vi "RIB - Shutdown.vi"(0 "Limits File Path":path, 5 "Results File Path":path, 11 "error in":errorcluster) -> (4 "Results Data Array":string[][](array[string]), 15 "error out":errorcluster)   [LabVIEW 2024]
doc: "Template test"
uses:
  <vilib>/addons/_JKI Toolkits/State Machine/_JKI_lib_State_Machine.llb/Select State(s)_err__jki_lib_state_machine.vi
  <vilib>/addons/_JKI Toolkits/State Machine/_JKI_lib_State_Machine.llb/Periodic Trigger__ogtk__JKI-SM__jki_lib_state_machine.vi
  <userlib>/_OpenG.lib/file/file.llb/Strip Path Extension - String__ogtk.vi
  <vilib>/Utility/file.llb/Read Delimited Spreadsheet (string).vi
  <userlib>/_OpenG.lib/appcontrol/appcontrol.llb/openg_application_control.lvlib
  <userlib>/_OpenG.lib/time/time.llb/openg_time.lvlib
  <userlib>/_OpenG.lib/file/file.llb/openg_file.lvlib
  I2C/libMPSSE-I2C.lvlib
  <vilib>/Utility/file.llb/Write Delimited Spreadsheet (string).vi
panel:
  in  "Exit":bool
  # "Shutdown"
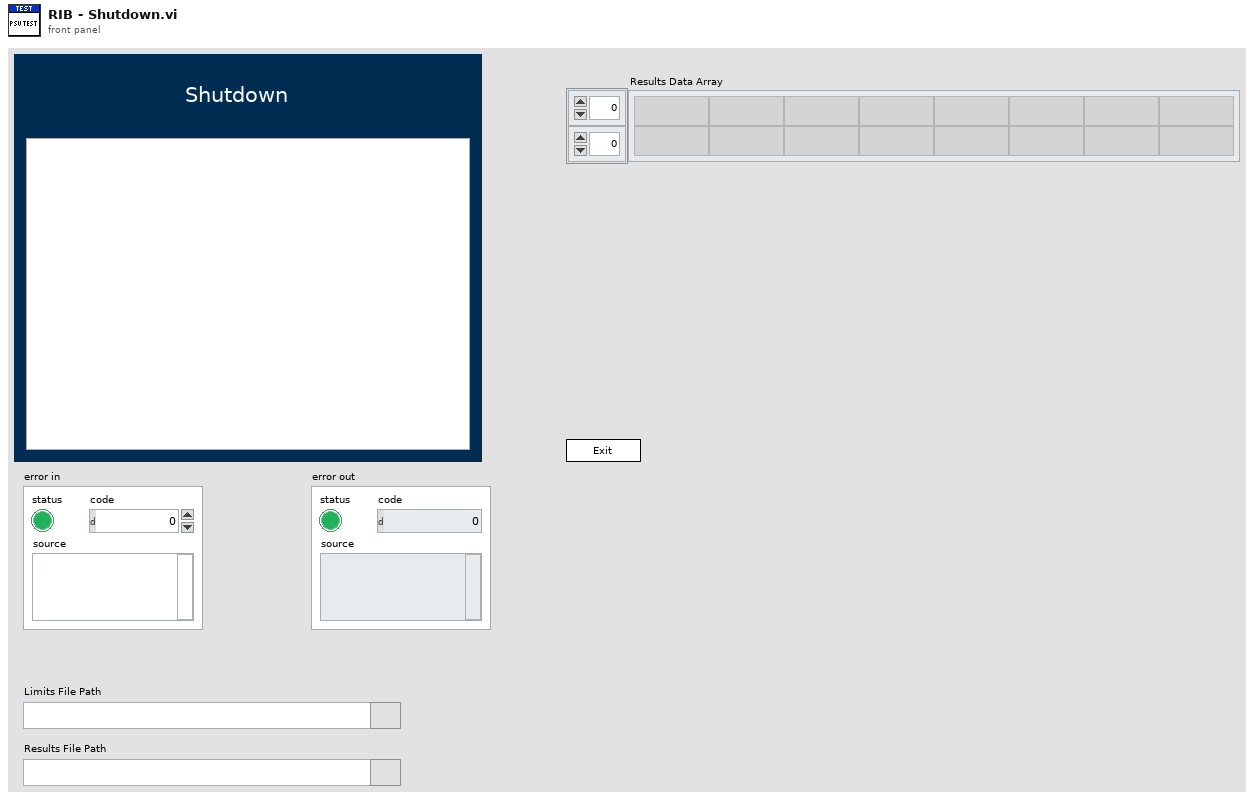
[diagram p1: front panel]
types:
  T1 = enum32{"Invalid", "Standard", "Closed", "Hidden", "Minimized", "Maximized"}
  T2 = enum32{"invalid app kind", "Development System", "Run Time System", "Student Edition", "Embedded LabVIEW", "Evaluation", "Custom"}
  T3 = typedef "FGV - Enum" = enum16{"Cleanup", "Get Data", "Open UDP", "Initialise DAQ", "Initialise I2C"}
  T4 = cluster{"Core":cluster{"Current VI Reference":refnum<vi>, "Close Panel on Exit?":bool}, "Limits File Path":path, "Test Limits":string[][], "Results Data Array":string[][], "Results File Path":path}
  T5 = cluster{"Current VI Reference":refnum<vi>, "Close Panel on Exit?":bool}
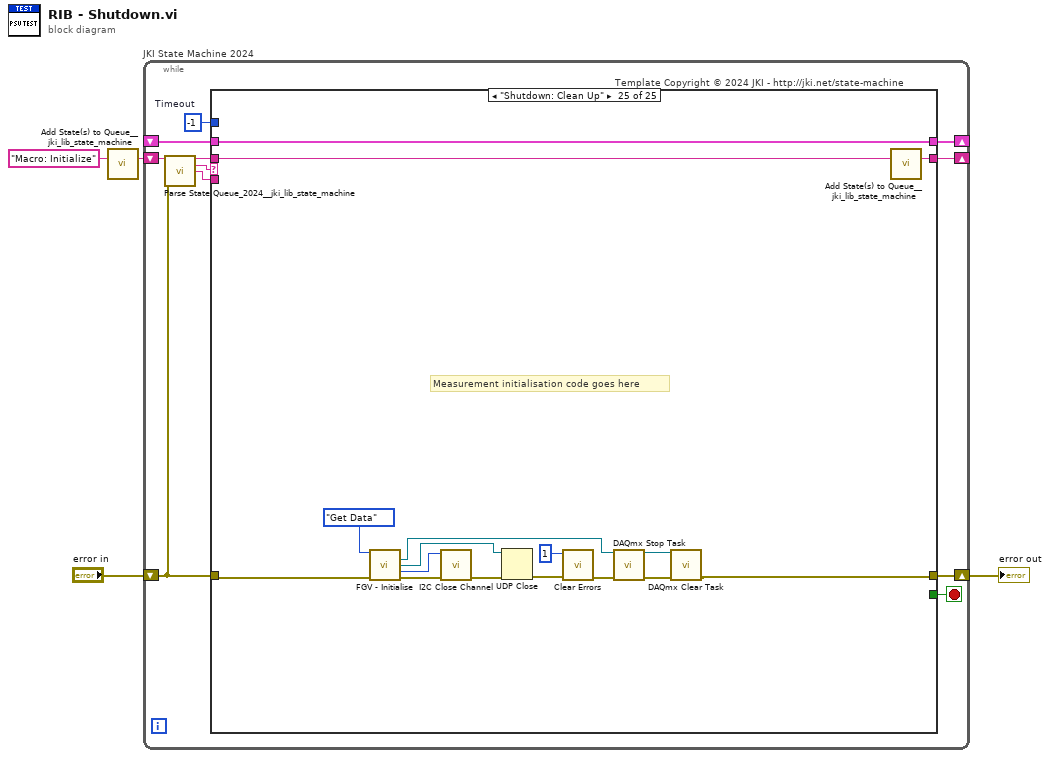
[diagram p0: block diagram]
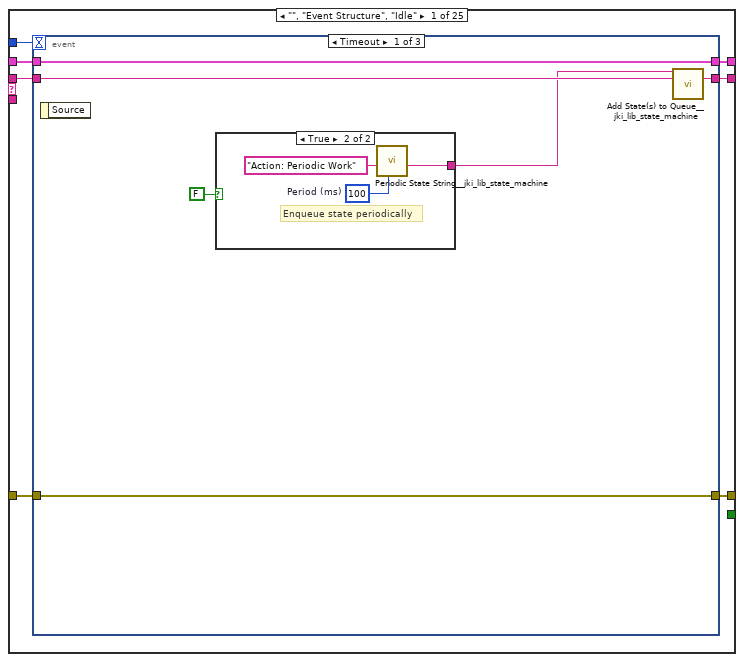
[diagram p2: hidden frame]
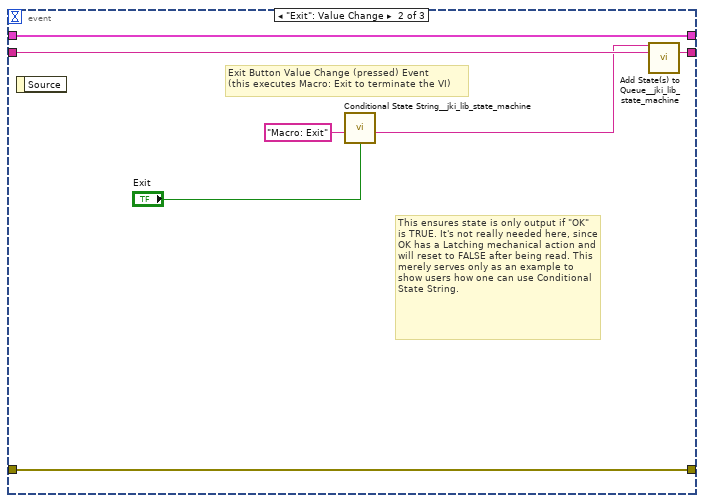
[diagram p4: hidden frame]
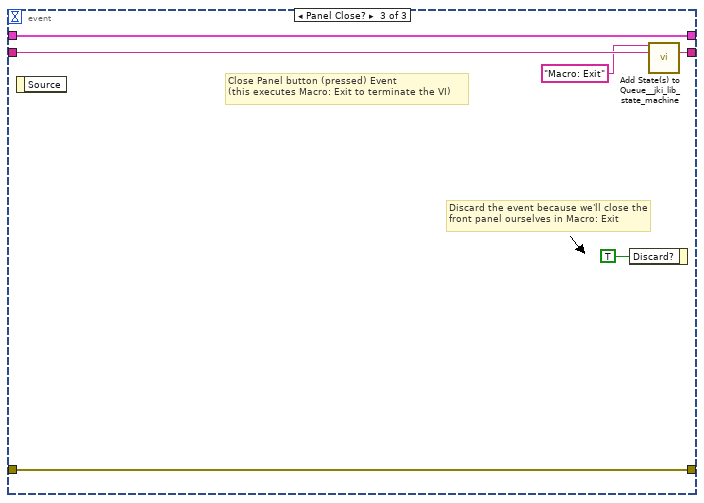
[diagram p5: hidden frame]
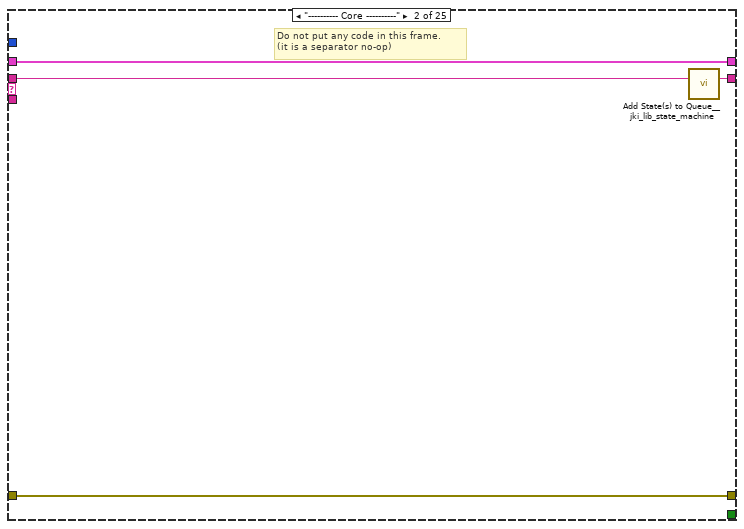
[diagram p6: hidden frame]
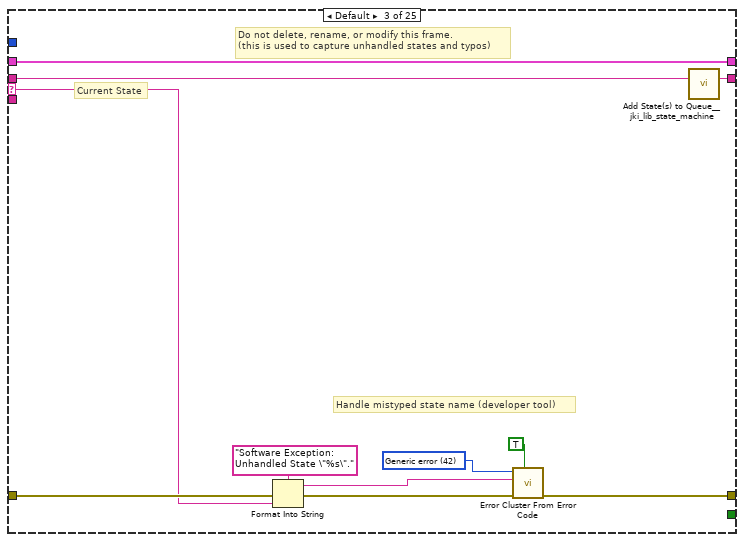
[diagram p7: hidden frame]
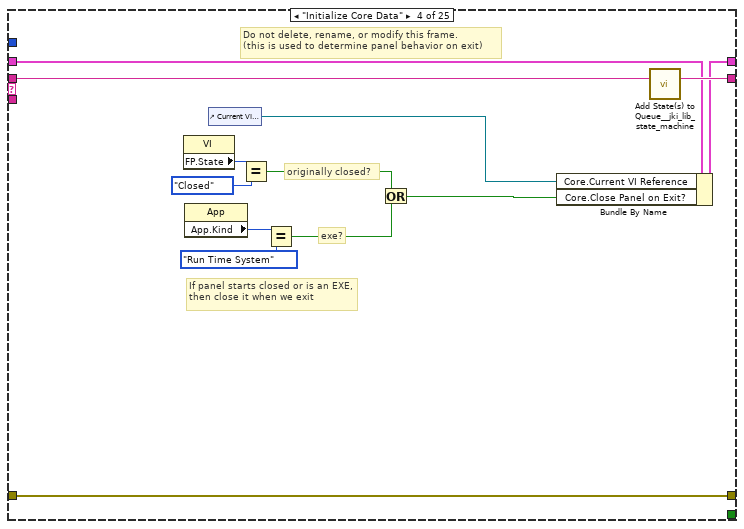
[diagram p8: hidden frame]
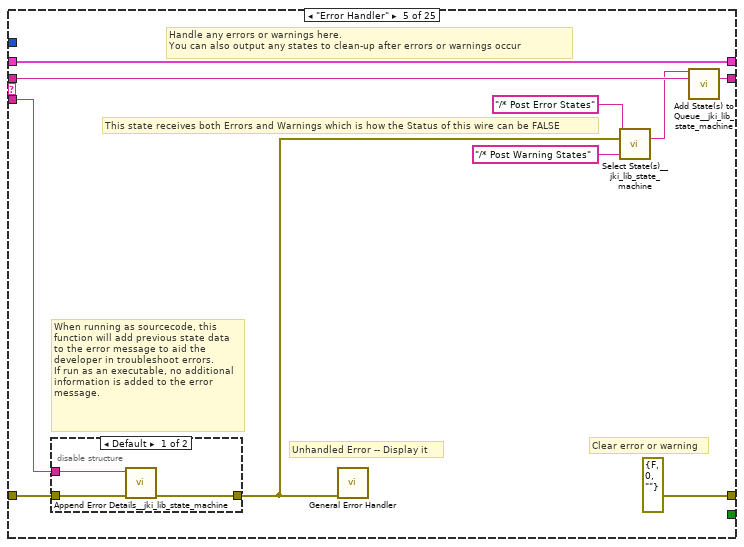
[diagram p9: hidden frame]
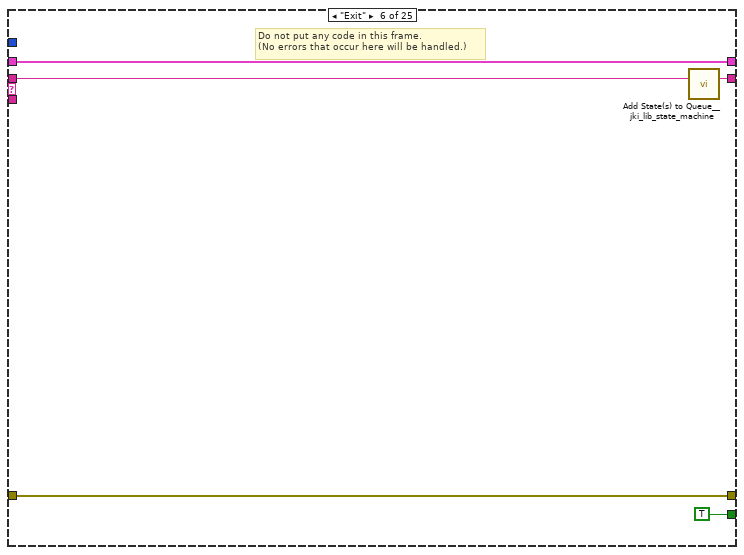
[diagram p11: hidden frame]
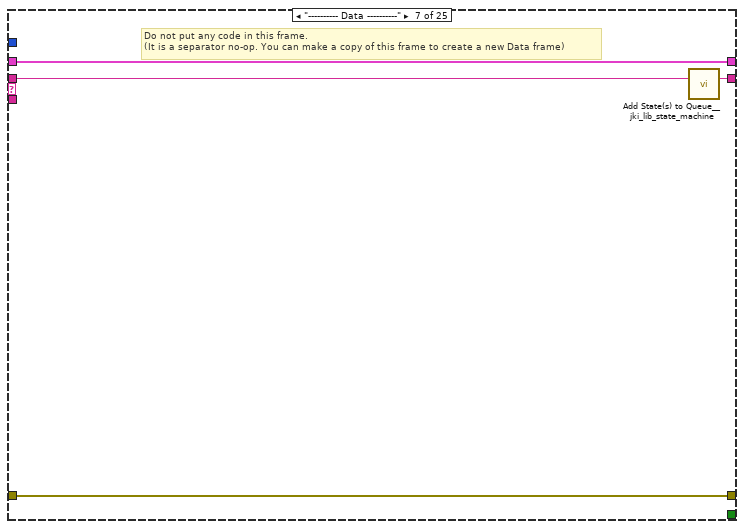
[diagram p12: hidden frame]
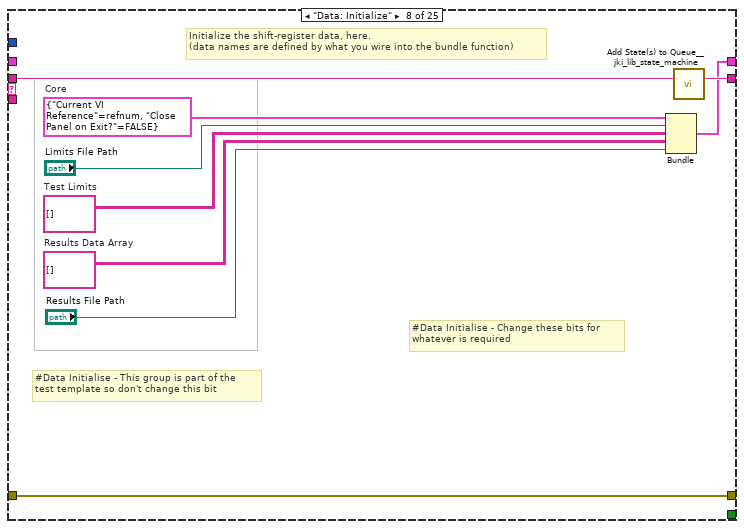
[diagram p13: hidden frame]
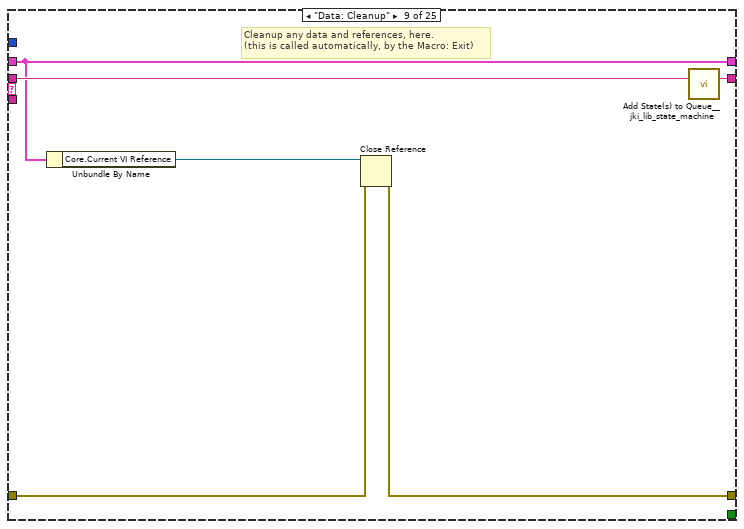
[diagram p14: hidden frame]
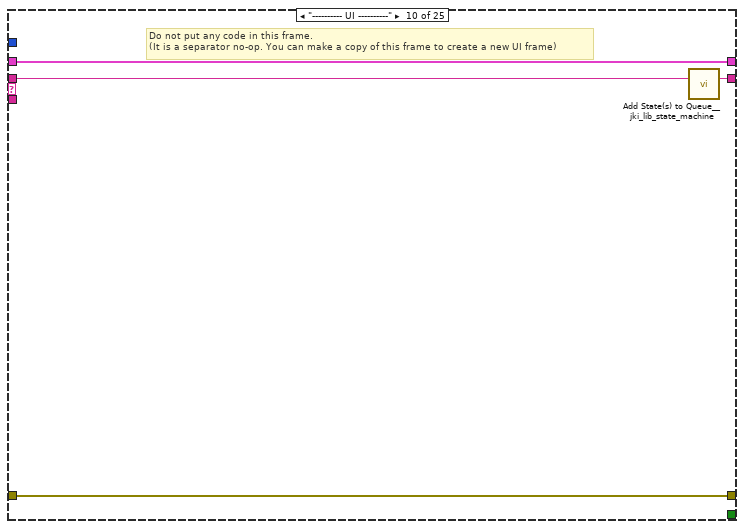
[diagram p15: hidden frame]
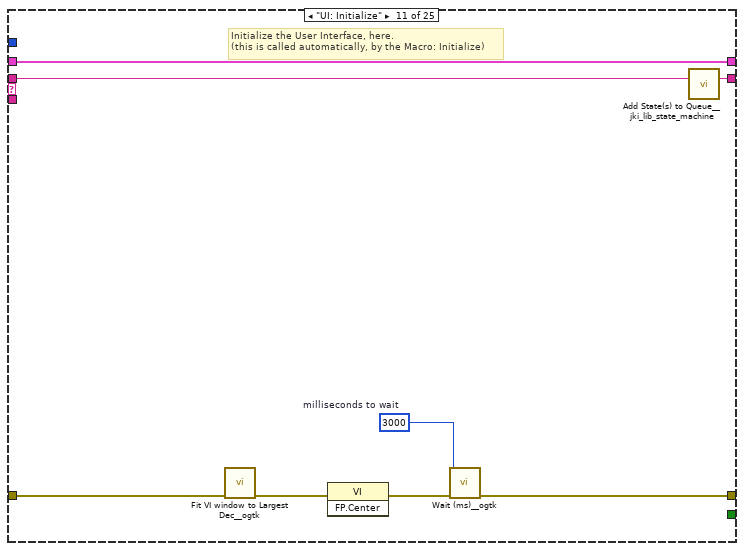
[diagram p16: hidden frame]
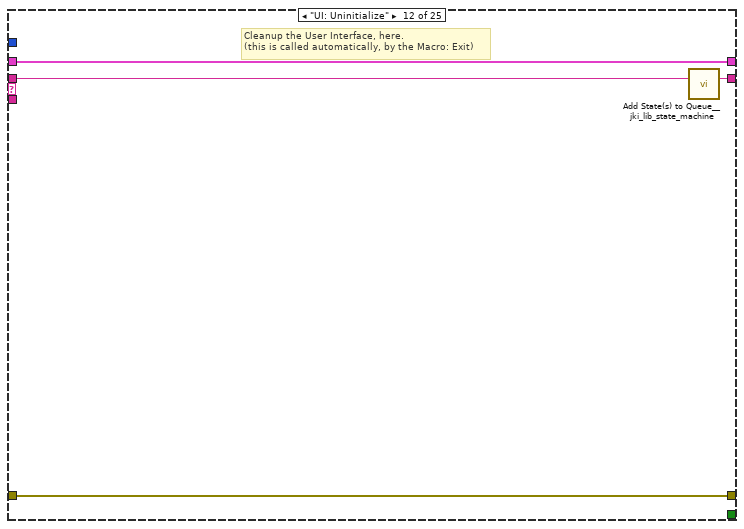
[diagram p17: hidden frame]
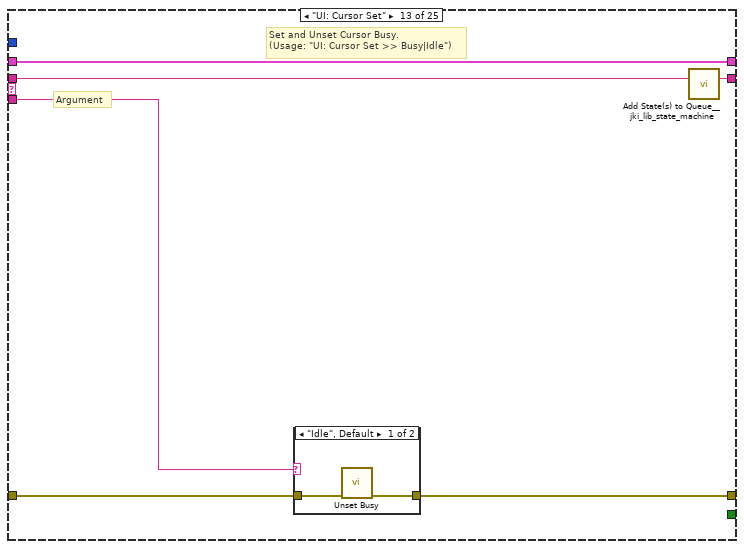
[diagram p18: hidden frame]
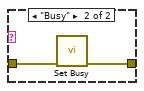
[diagram p19: hidden frame]
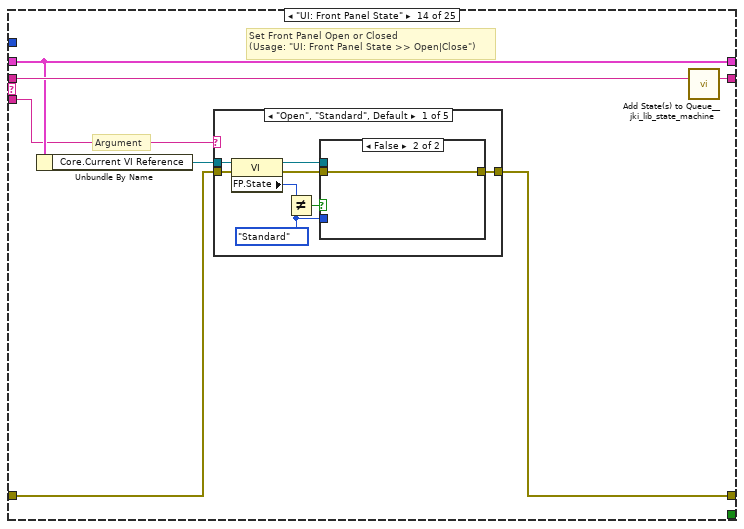
[diagram p20: hidden frame]
diagram:
  n1 = call <vilib>:"Add State(s) to Queue__jki_lib_state_machine.vi"("State(s) in (\"\")"="Macro: Initialize") -> ("States Out"=w4:string)  [unwired: 14 in]
  n2 = while "JKI State Machine 2024" {
    shift-right: [w8] -> _
    shift-left: _ -> [w7]
    shift-right: [w11] -> w1
    shift-left: "error in" -> [w5]
    shift-right: [w10] -> _
    shift-left: w4 -> [w12]
    stop <- w9 stop-if-true
    w6 = -1  # Timeout
    # "Template Copyright © 2024 JKI - http://jki.net/state-machine"
    n3 = call <vilib>:"Parse State Queue_2024__jki_lib_state_machine.vi"("State Queue"=w12, "Error In (no error)"=w5) -> ("Remaining States"=w14:string, "Current State"=w15:string, "Arguments"=w13:string)  [unwired: 11 in]
    n4 = case shown="\"Shutdown: Clean Up\"" w15 {
      selector: w15 -> [_ _ w49 _ _ _ _ _ _ _ _ _ _ _ _ _ _ _ _ _ _ _ _ _ _]
      tunnel: w14 -> [w22 w48 w53 w72 w82 w91 w95 w104 w110 w114 w122 w126 w132 w143 w212 w217 w221 w230 w234 w247 w257 w261 w270 w274 w290]
      tunnel: w13 -> [_ _ _ _ w77 _ _ _ _ _ _ _ w127 w137 _ _ _ _ _ _ _ _ _ _ _]
      tunnel: w7 -> [w20 w45 w51 w65 w79 w89 w92 _ w105 w111 w120 w124 w130 w139 w209 w214 w218 w228 w231 w237 w254 w259 w262 w271 w288]
      tunnel: [w19 w46 w55 w69 errorcluster {"status"=FALSE, "code"=0, "source"=""} ("error out") w88 w93 w101 w106 w112 w118 w123 w128 w140 w210 w215 w219 w225 w232 w235 w255 w258 w263 w272 w276] -> w11
      tunnel: w5 -> [w16 w46 w54 w69 w78 w88 w93 w101 w107 w112 w119 w123 w129 w141 w210 w215 w219 w225 w232 w236 w255 w258 w264 w272 w275]
      tunnel: [w21 w47 w52 w71 w81 w90 w94 w103 w109 w113 w121 w125 w131 w142 w211 w216 w220 w229 w233 w246 w256 w260 w269 w273 w289] -> w10
      tunnel: [_ _ _ _ _ TRUE _ _ _ _ _ _ _ _ _ _ _ _ _ _ _ _ _ _ _] -> w9
      tunnel: [w18 w45 w51 w70 w79 w89 w92 w102 w105 w111 w120 w124 w130 w139 w209 w214 w218 w228 w231 w238 w253 w259 w262 w271 w288] -> w8
      tunnel: w6 -> [w17 _ _ _ _ _ _ _ _ _ _ _ _ _ _ _ _ _ _ _ _ _ _ _ _]
      frame "", "Event Structure", "Idle" {
        n5 = event shown="[0] Timeout" {
          selector: _ -> [_ _ _]
          dyn-events: _ -> [_ _ _]
          timeout: w17 -> [_ _ _]
          tunnel: w22 -> [w28 w38 w44]
          tunnel: [w27 w37 w43] -> w21
          tunnel: w20 -> [w25 w35 w41]
          tunnel: [w26 w36 w42] -> w19
          tunnel: w16 -> [w26 w36 w42]
          tunnel: [w25 w35 w41] -> w18
          event Timeout {
            n6 = event-data() -> ()  [unwired: 1 in, 1 out]
            n7 = case shown="True" FALSE {
              tunnel: [_ w31] -> w24
              frame False {
              }
              frame True {
                w29 = u32 100  # Period (ms)
                # "Enqueue state periodically"
                n8 = call <vilib>:"Periodic State String__jki_lib_state_machine.vi"("Period (ms)"=w29, "State"="Action: Periodic Work") -> ("State Out"=w31:string)  [unwired: 9 in]
              }
            }
            n9 = call <vilib>:"Add State(s) to Queue__jki_lib_state_machine.vi"("State(s) in Front (\"\")"=w24, "State(s) in (\"\")"=w28) -> ("States Out"=w27:string)  [unwired: 13 in]
          }
          event "Exit": Value Change {
            # "This ensures state is only output if \"OK\" is TRUE. It's not really needed here, since OK has a Latching mechanical action and will reset to FALSE after being read. This merely serves only as an example to show users how one can use Conditional State String."
            # "Exit Button Value Change (pressed) Event\n(this executes Macro: Exit to terminate the VI)"
            n10 = event-data() -> ()  [unwired: 1 in, 1 out]
            n11 = call <vilib>:"Conditional State String__jki_lib_state_machine.vi"("Do State(s)?"="Exit", "State"="Macro: Exit") -> ("State Out"=w32:string)  [unwired: 7 in]
            n12 = call <vilib>:"Add State(s) to Queue__jki_lib_state_machine.vi"("State(s) in Front (\"\")"=w32, "State(s) in (\"\")"=w38) -> ("States Out"=w37:string)  [unwired: 13 in]
          }
          event Panel Close? {
            # "Discard the event because we'll close the front panel ourselves in Macro: Exit"
            # "Close Panel button (pressed) Event\n(this executes Macro: Exit to terminate the VI)"
            n13 = event-data() -> ()  [unwired: 1 in, 1 out]
            n14 = event-data("Discard?"=TRUE) -> ()  [unwired: 1 in, 1 out]
            n15 = call <vilib>:"Add State(s) to Queue__jki_lib_state_machine.vi"("State(s) in Front (\"\")"="Macro: Exit", "State(s) in (\"\")"=w44) -> ("States Out"=w43:string)  [unwired: 13 in]
          }
        }
      }
      frame "---------- Core ----------" {
        # "Do not put any code in this frame.\n(it is a separator no-op)"
        n16 = call <vilib>:"Add State(s) to Queue__jki_lib_state_machine.vi"("State(s) in (\"\")"=w48) -> ("States Out"=w47:string)  [unwired: 14 in]
      }
      frame Default {
        w58 = 42 items=["No error", "Argument error", "Memory is full", "Out of zone", "End of file", "File already open", "Generic file I/O error", "File not found", "File permission error", "Disk is full", "Duplicate path", "Too many files open", "System feature not enabled", "Resource file not found", "Cannot add resource", "Resource not found", "Image not found", "Image memory error", "Pen does not exist", "Config type invalid", "Config token not found", "Config parse error", "Config memory error", "Bad external code format", "Bad external code offset", "External code not present", "Null window", "Destroy window error", "Null menu", "Print aborted", "Bad print record", "Print driver error", "Windows error during printing", "Memory error during printing", "Print dialog error", "Generic print error", "Invalid device refnum", "Device not found", "Device parameter error", "Device unit error", "Cannot open device", "Device call aborted", "Generic error", "Cancelled by user", "Object ID too low", "Object ID too high", "Object not in heap", "Unknown heap", "Unknown object (invalid DefProc)", "Unknown object (DefProc not in table)", "Message out of range", "Invalid (null) method", "Unknown message", "Manager call not supported", "Bad address", "Network operation in progress", "Network operation timed out", "Connection is busy", "Network attribute not supported", "Network error", "Address in use", "System out of memory", "Connection aborted", "Connection refused", "Not connected", "Already connected", "Connection closed", "Initialization error (interapplication manager)", "Bad occurrence", "Wait on unbound occurrence handler", "Occurrence queue overflow", "Datalog type conflict", "Unused", "Unrecognized type (interapplication manager)", "Memory corrupt", "Failed to make temporary DLL", "Old CIN version", "Drag socket not found", "Failed to load drop-object", "Failed to register OLE object", "Failed to release OLE object", "Format specifier type mismatch", "Unknown format specifier", "Too few format specifiers", "Too many format specifiers", "Scan failed", "Newer CIN version", "Error converting to variant", "Runtime menu error", "Password tampered", "Variant attribute not found", "Incompatible variant data type", "Event data is not available", "Event Store is not present", "Occurrence is not found", "Event Queue is not created", "Event info is not available", "Refnum passed is NULL", "Error retrieving Class GUID", "Error retrieving CoClass GUID", "Error retrieving TypeLib GUID.", "Bad built application magic bytes.", "Specific driver is different from the specific driver associated with the Logical Name.", "There is no session opened to the class driver.", "Max Error", "MAX - Error with config objects", "MAX - Error loading configuration", "MAX - Group not supported"]
        # "Current State"
        # "Do not delete, rename, or modify this frame.\n(this is used to capture unhandled states and typos)"
        # "Handle mistyped state name (developer tool)"
        n17 = Format Into String(format string="Software Exception: Unhandled State \"%s\"." ("message"), error in=w54, w49) -> (resulting string=w57:string, error out=w56:errorcluster)  [unwired: 1 in]
        n18 = call <vilib>:"Error Cluster From Error Code.vi"("show call chain? (False)"=TRUE, "error in (no error)"=w56, "error message (\"\")"=w57, "error code (0)"=w58) -> ("error out"=w55:errorcluster)  [unwired: 5 in]
        n19 = call <vilib>:"Add State(s) to Queue__jki_lib_state_machine.vi"("State(s) in (\"\")"=w53) -> ("States Out"=w52:string)  [unwired: 14 in]
      }
      frame "Initialize Core Data" {
        # "Do not delete, rename, or modify this frame.\n(this is used to determine panel behavior on exit)"
        # "originally closed?"
        # "exe?"
        # "If panel starts closed or is an EXE, then close it when we exit"
        n20 = property class="VI"() -> ("FP.State"=w62:T1)  [unwired: 2 in, 2 out]
        n21 = property class="App"() -> ("App.Kind"=w68:T2)  [unwired: 2 in, 2 out]
        n22 = control-ref of="Current VI Reference"() -> (w63:refnum<vi>)
        n23 = Equal?(x=w62, y=T1."Closed" ("Front Panel Window:State")) -> (x = y?=w60:bool)
        n24 = Equal?(x=w68, y=T2."Run Time System" ("Application:Kind")) -> (x = y?=w66:bool)
        n25 = Or(x=w60, y=w66) -> (x .or. y?=w64:bool)
        n26 = Bundle By Name(cluster=w65, "Core.Current VI Reference"=w63, "Core.Close Panel on Exit?"=w64) -> (w70:T4)
        n27 = call <vilib>:"Add State(s) to Queue__jki_lib_state_machine.vi"("State(s) in (\"\")"=w72) -> ("States Out"=w71:string)  [unwired: 14 in]
      }
      frame "Error Handler" {
        # "When running as sourcecode, this function will add previous state data to the error message to aid the developer in troubleshoot errors.\nIf run as an executable, no additional information is added to the error message."
        # "This state receives both Errors and Warnings which is how the Status of this wire can be FALSE"
        # "Unhandled Error -- Display it"
        # "Handle any errors or warnings here.\nYou can also output any states to clean-up after errors or warnings occur"
        # "Clear error or warning"
        n28 = disable-structure shown="Default" {
          disable-tunnel: w78 -> [w85 w86]
          disable-tunnel: w77 -> [w84 _]
          disable-tunnel: [w83 w86] -> w76
          frame condition #0 (active) {
            n29 = call <vilib>:"Append Error Details__jki_lib_state_machine.vi"("error in (no error)"=w85, "Previous State and Argument(s)"=w84) -> ("error out"=w83:errorcluster)  [unwired: 9 in]
          }
          frame condition #1 {
          }
        }
        n30 = call <vilib>:"General Error Handler.vi"("error in (no error)"=w76) -> ()  [unwired: 10 in, 5 out]
        n31 = call-poly <vilib>:"Select State(s)__jki_lib_state_machine.vi"("State(s) if True (\"\")"="/* Post Error States", "Select"=w76, "State(s) if False (\"\")"="/* Post Warning States") -> ("States Out"=w74:string)  [unwired: 12 in]
        n32 = call <vilib>:"Add State(s) to Queue__jki_lib_state_machine.vi"("State(s) in Front (\"\")"=w74, "State(s) in (\"\")"=w82) -> ("States Out"=w81:string)  [unwired: 13 in]
      }
      frame "Exit" {
        # "Do not put any code in this frame.\n(No errors that occur here will be handled.)"
        n33 = call <vilib>:"Add State(s) to Queue__jki_lib_state_machine.vi"("State(s) in (\"\")"=w91) -> ("States Out"=w90:string)  [unwired: 14 in]
      }
      frame "---------- Data ----------" {
        # "Do not put any code in this frame.\n(It is a separator no-op. You can make a copy of this frame to create a new Data frame)"
        n34 = call <vilib>:"Add State(s) to Queue__jki_lib_state_machine.vi"("State(s) in (\"\")"=w95) -> ("States Out"=w94:string)  [unwired: 14 in]
      }
      frame "Data: Initialize" {
        w97 = string[][] []  # Results Data Array
        w98 = string[][] []  # Test Limits
        w100 = T5 {"Current VI Reference"=refnum, "Close Panel on Exit?"=FALSE}  # Core
        # "#Data Initialise - Change these bits for\nwhatever is required"
        # "#Data Initialise - This group is part of the\ntest template so don't change this bit"
        # "Initialize the shift-register data, here.\n(data names are defined by what you wire into the bundle function)"
        n35 = Bundle("Core"=w100, "Limits File Path"="Limits File Path", "Test Limits"=w98, "Results Data Array"=w97, "Results File Path"="Results File Path") -> (w102:T4)  [unwired: 1 in]
        n36 = call <vilib>:"Add State(s) to Queue__jki_lib_state_machine.vi"("State(s) in (\"\")"=w104) -> ("States Out"=w103:string)  [unwired: 14 in]
      }
      frame "Data: Cleanup" {
        # "Cleanup any data and references, here.\n(this is called automatically, by the Macro: Exit)"
        n37 = Unbundle By Name(w105) -> ("Core.Current VI Reference"=w108:refnum<vi>)
        n38 = Close Reference(reference=w108, error in (no error)=w107) -> (error out=w106:errorcluster)
        n39 = call <vilib>:"Add State(s) to Queue__jki_lib_state_machine.vi"("State(s) in (\"\")"=w110) -> ("States Out"=w109:string)  [unwired: 14 in]
      }
      frame "---------- UI ----------" {
        # "Do not put any code in this frame.\n(It is a separator no-op. You can make a copy of this frame to create a new UI frame)"
        n40 = call <vilib>:"Add State(s) to Queue__jki_lib_state_machine.vi"("State(s) in (\"\")"=w114) -> ("States Out"=w113:string)  [unwired: 14 in]
      }
      frame "UI: Initialize" {
        w117 = u32 3000  # milliseconds to wait
        # "Initialize the User Interface, here.\n(this is called automatically, by the Macro: Initialize)"
        n41 = call <userlib>:"Fit VI window to Largest Dec__ogtk.vi"("error in (no error)"=w119) -> ("error out"=w115:errorcluster)  [unwired: 5 in, 1 out]
        n42 = invoke class="VI" method="FP.Center"(error in=w115) -> (error out=w116:errorcluster)  [unwired: 2 in, 2 out]
        n43 = call <userlib>:"Wait (ms)__ogtk.vi"("error in (no error)"=w116, "milliseconds to wait"=w117) -> ("error out"=w118:errorcluster)  [unwired: 8 in, 1 out]
        n44 = call <vilib>:"Add State(s) to Queue__jki_lib_state_machine.vi"("State(s) in (\"\")"=w122) -> ("States Out"=w121:string)  [unwired: 14 in]
      }
      frame "UI: Uninitialize" {
        # "Cleanup the User Interface, here.\n(this is called automatically, by the Macro: Exit)"
        n45 = call <vilib>:"Add State(s) to Queue__jki_lib_state_machine.vi"("State(s) in (\"\")"=w126) -> ("States Out"=w125:string)  [unwired: 14 in]
      }
      frame "UI: Cursor Set" {
        # "Argument"
        # "Set and Unset Cursor Busy.\n(Usage: \"UI: Cursor Set >> Busy|Idle\")"
        n46 = case shown="\"Idle\", Default" w127 {
          tunnel: w129 -> [w134 w136]
          tunnel: [w133 w135] -> w128
          frame "Idle", Default {
            n47 = call <vilib>:"Unset Busy.vi"("error in (no error)"=w134) -> ("error out"=w133:errorcluster)  [unwired: 10 in]
          }
          frame "Busy" {
            n48 = call <vilib>:"Set Busy.vi"("error in (no error)"=w136) -> ("error out"=w135:errorcluster)  [unwired: 9 in, 1 out]
          }
        }
        n49 = call <vilib>:"Add State(s) to Queue__jki_lib_state_machine.vi"("State(s) in (\"\")"=w132) -> ("States Out"=w131:string)  [unwired: 14 in]
      }
      frame "UI: Front Panel State" {
        # "Argument"
        # "Set Front Panel Open or Closed\n(Usage: \"UI: Front Panel State >> Open|Close\")"
        n50 = Unbundle By Name(w139) -> ("Core.Current VI Reference"=w138:refnum<vi>)
        n51 = case shown="\"Open\", \"Standard\", Default" w137 {
          tunnel: w141 -> [w149 w164 w175 w188 w201]
          tunnel: [w151 w165 w177 w190 w203] -> w140
          tunnel: w138 -> [w150 w162 w176 w189 w202]
          frame "Open", "Standard", Default {
            w144 = T1."Standard" ("State")
            n52 = property class="VI"(reference=w150, error in=w149) -> (reference out=w147:refnum<vi>, error out=w148:errorcluster, "FP.State"=w146:T1)
            n53 = Not Equal?(x=w146, y=w144) -> (x != y?=w145:bool)
            n54 = case shown="False" w145 {
              tunnel: [w155 w157] -> w151
              tunnel: w148 -> [w154 w157]
              tunnel: w147 -> [w153 _]
              tunnel: w144 -> [w152 _]
              frame True {
                n55 = invoke class="VI" method="FP.Open"(reference=w153, error in=w154, "Activate"=TRUE, "State"=w152) -> (error out=w155:errorcluster)  [unwired: 1 in, 4 out]
              }
              frame False {
              }
            }
          }
          frame "Close", "Closed" {
            n56 = property class="VI"(reference=w162, error in=w164) -> (reference out=w161:refnum<vi>, error out=w163:errorcluster, "FP.State"=w159:T1)
            n57 = Not Equal?(x=w159, y=T1."Closed" ("Front Panel Window:State")) -> (x != y?=w158:bool)
            n58 = case shown="True" w158 {
              tunnel: [w166 w169] -> w165
              tunnel: w163 -> [w166 w168]
              tunnel: w161 -> [_ w167]
              frame False {
              }
              frame True {
                n59 = invoke class="VI" method="FP.Close"(reference=w167, error in=w168) -> (error out=w169:errorcluster)  [unwired: 1 in, 2 out]
              }
            }
          }
          frame "Hidden", "Hide" {
            w170 = T1."Hidden" ("State")
            n60 = property class="VI"(reference=w176, error in=w175) -> (reference out=w173:refnum<vi>, error out=w174:errorcluster, "FP.State"=w172:T1)
            n61 = Not Equal?(x=w172, y=w170) -> (x != y?=w171:bool)
            n62 = case shown="True" w171 {
              tunnel: [w181 w182] -> w177
              tunnel: w174 -> [w180 w182]
              tunnel: w173 -> [w179 _]
              tunnel: w170 -> [w178 _]
              frame True {
                n63 = invoke class="VI" method="FP.Open"(reference=w179, error in=w180, "State"=w178) -> (error out=w181:errorcluster)  [unwired: 2 in, 4 out]
              }
              frame False {
              }
            }
          }
          frame "Minimize", "Minimized" {
            w183 = T1."Minimized" ("State")
            n64 = property class="VI"(reference=w189, error in=w188) -> (reference out=w186:refnum<vi>, error out=w187:errorcluster, "FP.State"=w185:T1)
            n65 = Not Equal?(x=w185, y=w183) -> (x != y?=w184:bool)
            n66 = case shown="True" w184 {
              tunnel: [w194 w195] -> w190
              tunnel: w187 -> [w193 w195]
              tunnel: w186 -> [w192 _]
              tunnel: w183 -> [w191 _]
              frame True {
                n67 = invoke class="VI" method="FP.Open"(reference=w192, error in=w193, "State"=w191) -> (error out=w194:errorcluster)  [unwired: 2 in, 4 out]
              }
              frame False {
              }
            }
          }
          frame "Maximize", "Maximized" {
            w196 = T1."Maximized" ("State")
            n68 = property class="VI"(reference=w202, error in=w201) -> (reference out=w199:refnum<vi>, error out=w200:errorcluster, "FP.State"=w198:T1)
            n69 = Not Equal?(x=w198, y=w196) -> (x != y?=w197:bool)
            n70 = case shown="True" w197 {
              tunnel: [w207 w208] -> w203
              tunnel: w200 -> [w206 w208]
              tunnel: w199 -> [w205 _]
              tunnel: w196 -> [w204 _]
              frame True {
                n71 = invoke class="VI" method="FP.Open"(reference=w205, error in=w206, "State"=w204) -> (error out=w207:errorcluster)  [unwired: 2 in, 4 out]
              }
              frame False {
              }
            }
          }
        }
        n72 = call <vilib>:"Add State(s) to Queue__jki_lib_state_machine.vi"("State(s) in (\"\")"=w143) -> ("States Out"=w142:string)  [unwired: 14 in]
      }
      frame "---------- Macro ----------" {
        # "Do not put any code in this frame.\n(It is a separator no-op. You can make a copy of this frame to create a new Macro frame)"
        n73 = call <vilib>:"Add State(s) to Queue__jki_lib_state_machine.vi"("State(s) in (\"\")"=w212) -> ("States Out"=w211:string)  [unwired: 14 in]
      }
      frame "Macro: Initialize" {
        # "Initialization Macro\n(This is called once, when the VI starts)"
        n74 = call <vilib>:"Add State(s) to Queue__jki_lib_state_machine.vi"("State(s) in Front (\"\")"="Data: Initialize\nInitialize Core Data\nLimits Test: Read Limits File\nLimits Test: Test\nResults Data: Write Results Data\nUI: Initialize\nUI: Front Panel State >> Open\nShutdown: Clean Up\nMacro: Exit", "State(s) in (\"\")"=w217) -> ("States Out"=w216:string)  [unwired: 13 in]
      }
      frame "Macro: Test" {
        (unwired) "Macro: Exit"
        # "#Test Macro - Add the sequence \nfor measurments and limits testing here"
        n75 = call <vilib>:"Add State(s) to Queue__jki_lib_state_machine.vi"("State(s) in (\"\")"=w221) -> ("States Out"=w220:string)  [unwired: 14 in]
      }
      frame "Macro: Exit" {
        # "Exit Macro\n(This is called once, when the VI exits)"
        n76 = Unbundle By Name(w228) -> ("Core.Close Panel on Exit?"=w223:bool)
        n77 = call <vilib>:"Conditional State String__jki_lib_state_machine.vi"("Do State(s)?"=w223, "State"="UI: Front Panel State >> Close") -> ("State Out"=w222:string)  [unwired: 7 in]
        n78 = call <vilib>:"Add State(s) to Queue__jki_lib_state_machine.vi"("State(s) in (\"\")"=w222, "State(s) at Back (\"\")"="UI: Uninitialize\nData: Cleanup\nLimits Test: Test\nExit") -> ("States Out"=w226:string)  [unwired: 13 in]
        n79 = call <vilib>:"Add State(s) to Queue__jki_lib_state_machine.vi"("State(s) in Front (\"\")"=w226, "State(s) in (\"\")"=w230) -> ("States Out"=w229:string)  [unwired: 13 in]
      }
      frame "---------- Limits Test ----------" {
        # "Do not put any code in this frame.\n(It is a separator no-op. You can make a copy of this frame to create a new UI frame)"
        n80 = call <vilib>:"Add State(s) to Queue__jki_lib_state_machine.vi"("State(s) in (\"\")"=w234) -> ("States Out"=w233:string)  [unwired: 14 in]
      }
      frame "Limits Test: Read Limits File" {
        w242 = ","  # delimiter (\t)
        # "Do not put any code in this frame.\n(It is a separator no-op. You can make a copy of this frame to create a new UI frame)"
        n81 = Unbundle By Name(w237) -> ("Limits File Path"=w243:path)
        n82 = Current VI's Path "Test Case Path"() -> (path=w245:path)
        n83 = call-poly <vilib>:"Read Delimited Spreadsheet.vi"("file path (dialog if empty)"=w243, "error in (no error)"=w236, "delimiter (\\t)"=w242) -> ("all rows"=w240:string[][], "error out"=w235:errorcluster)  [unwired: 7 in, 4 out]
        n84 = Strip Path(path=w245) -> (name=w244:string)  [unwired: 1 out]
        n85 = call-poly <userlib>:"Strip Path Extension__ogtk.vi"("path"=w244) -> ("root"=w241:string)  [unwired: 1 out]
        n86 = for {
          tunnel: w241 -> [w251]
          tunnel: w240 -> [w249] mode=indexing
          tunnel: [w249] -> w239 mode=indexing if=w248
          n87 = Index Array(array=w249) -> (element=w250:string)  [unwired: 1 in]
          n88 = Equal?(x=w251, y=w250) -> (x = y?=w248:bool)
        }
        n89 = Bundle By Name(cluster=w237, "Test Limits"=w239) -> (w238:T4)
        n90 = call <vilib>:"Add State(s) to Queue__jki_lib_state_machine.vi"("State(s) in (\"\")"=w247) -> ("States Out"=w246:string)  [unwired: 14 in]
      }
      frame "Limits Test: Test" {
        # "Do not put any code in this frame.\n(It is a separator no-op. You can make a copy of this frame to create a new UI frame)"
        n91 = Bundle By Name(cluster=w254, "Results Data Array"=string[][] [["Shutdown", "Clean Up", "Action", "", "", "", "", "Passed"]]) -> (w253:T4)
        n92 = call <vilib>:"Add State(s) to Queue__jki_lib_state_machine.vi"("State(s) in (\"\")"=w257) -> ("States Out"=w256:string)  [unwired: 14 in]
      }
      frame "---------- Results Data ----------" {
        # "Do not put any code in this frame.\n(It is a separator no-op. You can make a copy of this frame to create a new UI frame)"
        n93 = call <vilib>:"Add State(s) to Queue__jki_lib_state_machine.vi"("State(s) in (\"\")"=w261) -> ("States Out"=w260:string)  [unwired: 14 in]
      }
      frame "Results Data: Write Results Data" {
        w266 = ","  # delimiter (\t)
        w267 = TRUE  # append to file? (new file:F)
        # "Do not put any code in this frame.\n(It is a separator no-op. You can make a copy of this frame to create a new UI frame)"
        n94 = Unbundle By Name(w262) -> ("Results File Path"=w268:path, "Results Data Array"=w265:string[][])
        "Results Data Array" <- w265
        n95 = call-poly <vilib>:"Write Delimited Spreadsheet.vi"("file path (dialog if empty)"=w268, "2D data"=w265, "append to file? (new file:F)"=w267, "error in (no error)"=w264, "delimiter (\\t)"=w266) -> ("error out"=w263:errorcluster)  [unwired: 9 in, 1 out]
        n96 = call <vilib>:"Add State(s) to Queue__jki_lib_state_machine.vi"("State(s) in (\"\")"=w270) -> ("States Out"=w269:string)  [unwired: 14 in]
      }
      frame "---------- Shutdown ----------" {
        # "Template Separator\n(You can make a copy of, or modify, this frame)"
        n97 = call <vilib>:"Add State(s) to Queue__jki_lib_state_machine.vi"("State(s) in (\"\")"=w274) -> ("States Out"=w273:string)  [unwired: 14 in]
      }
      frame "Shutdown: Clean Up" {
        # "Measurement initialisation code goes here"
        n98 = call "FGV - Initialise.vi"("Enum"=FGV_-_Enum."Get Data", "Error In"=w275) -> ("task out"=w281:refnum<k21>, "connection ID"=w282:refnum<k16>, "Handle Out"=w283:u64, "Error Out"=w284:errorcluster)  [unwired: 10 in]
        n99 = call "I2C Close Channel.vi"("error in (no error)"=w284, "handle"=w283) -> ("error out"=w280:errorcluster)  [unwired: 7 in, 2 out]
        n100 = UDP Close(connection ID=w282, 8:w280) -> (error out=w279:errorcluster)  [unwired: 1 out]
        n101 = call <vilib>:"Clear Errors.vi"("error in (no error)"=w279, "specific error code to clear (0: all)"=1) -> ("error out"=w278:errorcluster)  [unwired: 4 in, 1 out]
        n102 = call <vilib>:"DAQmx Stop Task.vi"("task/channels in"=w281, "error in"=w278) -> ("task out"=w286:refnum<k21>, "error out"=w287:errorcluster)  [unwired: 12 in]
        n103 = call <vilib>:"DAQmx Clear Task.vi"("task in"=w286, "error in"=w287) -> ("error out"=w276:errorcluster)  [unwired: 13 in]
        n104 = call <vilib>:"Add State(s) to Queue__jki_lib_state_machine.vi"("State(s) in (\"\")"=w290) -> ("States Out"=w289:string)  [unwired: 14 in]
      }
    }
  }
  "error out" <- w1
